vi "Vi_ExecutionDesSequences.vi"(6 "Acceleration":dbl, 7 "Deceleration":dbl, 9 "Axe":i32=1, 10 "Vitesse":dbl, 11 "Angle":dbl) -> (0 "Deverouillé":bool, 8 "Connecté":bool)   [LabVIEW 2015]
uses:
  Variable globale.vi
  <userlib>/ICNC/ICNC2.lvlib
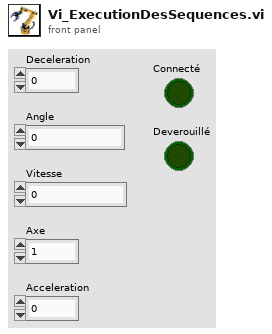
[diagram p1: front panel]
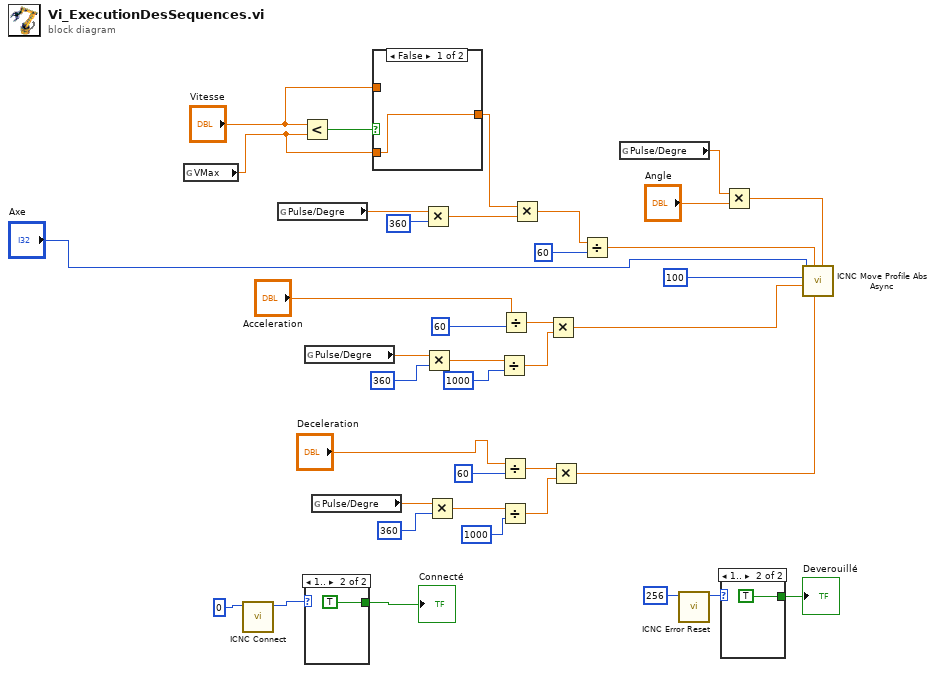
[diagram p0: block diagram]
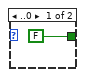
[diagram p2: hidden frame]
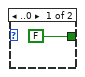
[diagram p3: hidden frame]
diagram:
  n1 = global read "Variable globale.vi" "VMax"() -> (w27:dbl)
  n2 = call <userlib>:"ICNC Connect.vi"("ICNC_Number"=0) -> ("function return"=w4:u32)  [unwired: 9 in, 1 out]
  n3 = global read "Variable globale.vi" "Pulse/Degre"() -> (w18:dbl)
  n4 = Less?(x="Vitesse", y=w27) -> (x < y?=w25:bool)
  n5 = global read "Variable globale.vi" "Pulse/Degre"() -> (w9:dbl)
  n6 = case shown="1.." w4 {
    tunnel: [FALSE TRUE] -> w1
    frame ..0 {
    }
    frame 1.. {
    }
  }
  "Connecté" <- w1
  n7 = global read "Variable globale.vi" "Pulse/Degre"() -> (w15:dbl)
  n8 = case shown="False" w25 {
    tunnel: "Vitesse" -> [_ w43]
    tunnel: w27 -> [w42 _]
    tunnel: [w42 w43] -> w31
    frame False {
    }
    frame True {
    }
  }
  n9 = Multiply(x=w18, y=360) -> (x*y=w30:dbl)
  n10 = Multiply(x=w9, y=360) -> (x*y=w28:dbl)
  n11 = Multiply(x=w15, y=360) -> (x*y=w29:dbl)
  n12 = Divide(x=w28, y=1000) -> (x/y=w8:dbl)
  n13 = Divide(x="Deceleration", y=60) -> (x/y=w13:dbl)
  n14 = Divide(x=w29, y=1000) -> (x/y=w14:dbl)
  n15 = Divide(x="Acceleration", y=60) -> (x/y=w21:dbl)
  n16 = Multiply(x=w31, y=w30) -> (x*y=w22:dbl)
  n17 = Multiply(x=w21, y=w8) -> (x*y=w35:dbl)
  n18 = Multiply(x=w13, y=w14) -> (x*y=w36:dbl)
  n19 = Divide(x=w22, y=60) -> (x/y=w33:dbl)
  n20 = global read "Variable globale.vi" "Pulse/Degre"() -> (w23:dbl)
  n21 = call <userlib>:"ICNC Error Reset.vi"("ErrorBits"=256) -> ("function return"=w5:u32)  [unwired: 9 in, 1 out]
  n22 = case shown="1.." w5 {
    tunnel: [FALSE TRUE] -> w2
    frame ..0 {
    }
    frame 1.. {
    }
  }
  "Deverouillé" <- w2
  n23 = Multiply(x=w23, y="Angle") -> (x*y=w32:dbl)
  n24 = call <userlib>:"ICNC Move Profile Abs Async.vi"("Position"=w32, "Decel"=w36, "Speed"=w33, "Accel"=w35, "FStartStop"=100, "Axe"="Axe") -> ()  [unwired: 4 in, 2 out]
